vi "PreCalc FDFrame Durations.vi"(8 "error in (no error)":errorcluster, 9 "Bit Time FD (seconds)":dbl, 10 "Bit Time (seconds)":dbl, 11 "CANBus_Load_Calculator in":refnum<class "CANBus_Load_Calculator.lvclass">) -> (0 "error out":errorcluster, 3 "CANBus_Load_Calculator out":refnum<class "CANBus_Load_Calculator.lvclass">)   [LabVIEW 2018, in "NI-XNET Monitor Engine.lvlib" / "XNET-Bus-Load-Calculator.lvlib" / "CANBus_Load_Calculator.lvclass"]
uses:
  CANBus_Load_Calculator.lvclass
  typedefs/CANFD_Frame_Timing.ctl
  CANBus_Load_Calculator.lvclass/CANBus_Load_Calculator.ctl
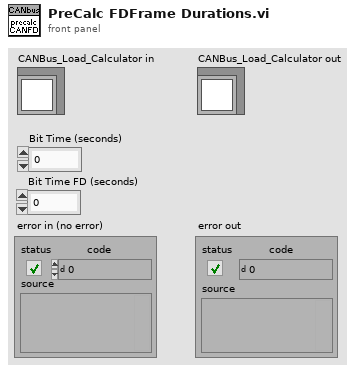
[diagram p1: front panel]
types:
  T1 = typedef "NI-XNET Monitor Engine.lvlib/XNET-Bus-Load-Calculator.lvlib/CANBus_Load_Calculator.lvclass/CANFD_Frame_Timing.ctl" = cluster{"Frame Length (Bytes)":i32, "FD.StdID.AvgDuration (us)":u32, "FD.ExtID.AvgDuration (us)":u32, "FDBRS.StdID.AvgDuration (us)":u32, "FDBRS.ExtID.AvgDuration (us)":u32}
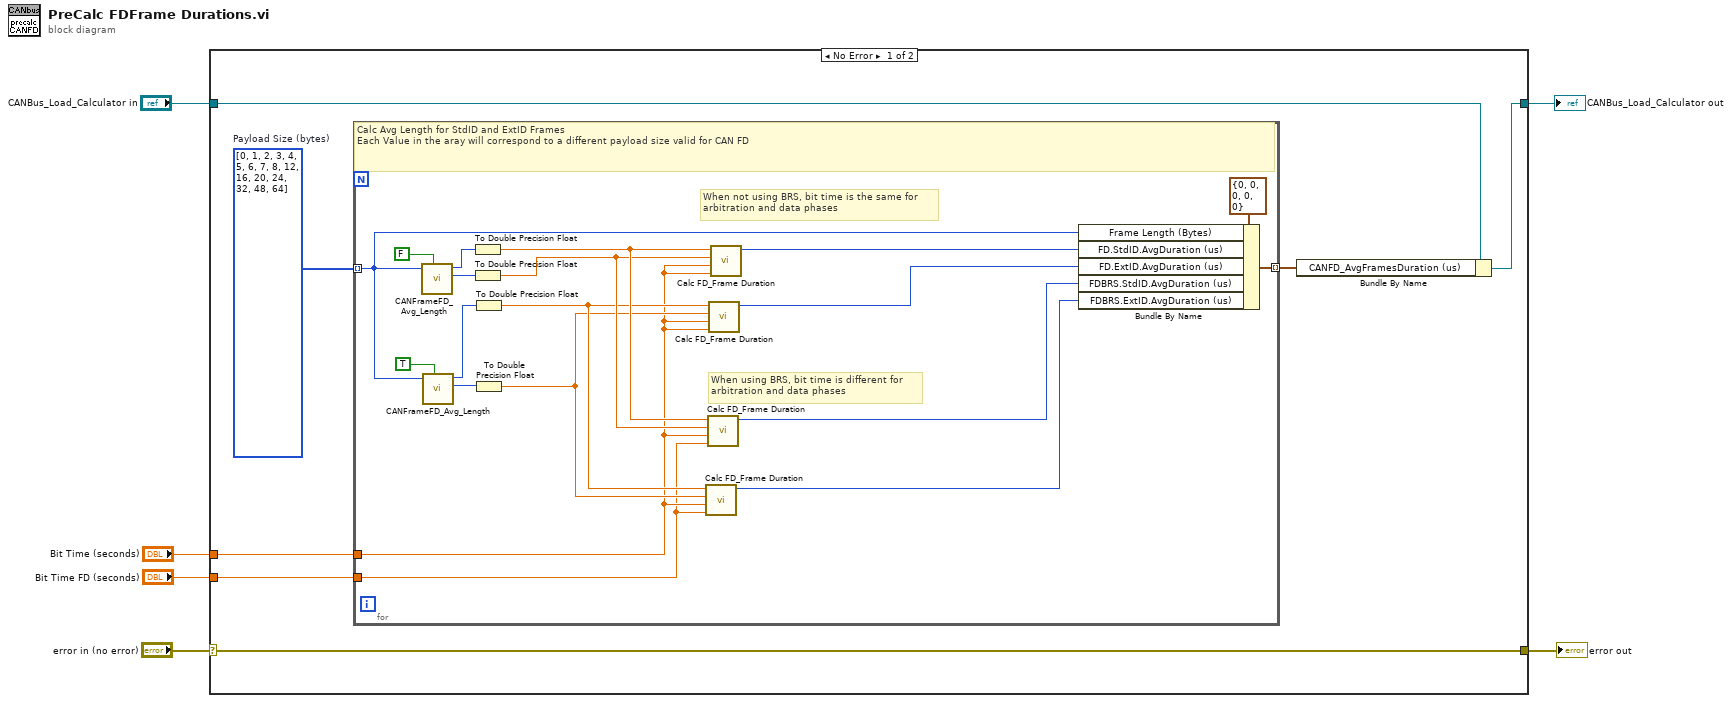
[diagram p0: block diagram]
diagram:
  n1 = case shown="No Error" "error in (no error)" {
    selector: "error in (no error)" -> [w11 w34]
    tunnel: "Bit Time (seconds)" -> [w9 _]
    tunnel: [w13 w33] -> w5
    tunnel: "CANBus_Load_Calculator in" -> [w12 w33]
    tunnel: [w11 w34] -> w2
    tunnel: "Bit Time FD (seconds)" -> [w8 _]
    frame No Error {
      w10 = i32[] [0, 1, 2, 3, 4, 5, 6, 7, 8, 12, 16, 20, 24, 32, 48, 64]  # Payload Size (bytes)
      n2 = for {
        tunnel: w10 -> [w28] mode=indexing
        tunnel: w9 -> [w15]
        tunnel: w8 -> [w14]
        tunnel: [w29] -> w7 mode=indexing
        # "When not using BRS, bit time is the same for\narbitration and data phases"
        # "When using BRS, bit time is different for\narbitration and data phases"
        # "Calc Avg Length for StdID and ExtID Frames\nEach Value in the aray will correspond to a different payload size valid for CAN FD"
        n3 = call "CANFrameFD_Avg_Length.vi"("Payload Size (bytes)"=w28, "Extended ID?"=FALSE) -> ("Avg.ArbitrationLength (bits)"=w27:i32, "Avg.DataLength (bits)"=w26:i32)  [unwired: 5 in]
        n4 = call "CANFrameFD_Avg_Length.vi"("Payload Size (bytes)"=w28, "Extended ID?"=TRUE) -> ("Avg.ArbitrationLength (bits)"=w25:i32, "Avg.DataLength (bits)"=w24:i32)  [unwired: 5 in]
        n5 = To Double Precision Float(number=w27) -> (double precision float=w21:dbl)
        n6 = To Double Precision Float(number=w26) -> (double precision float=w20:dbl)
        n7 = To Double Precision Float(number=w25) -> (double precision float=w19:dbl)
        n8 = To Double Precision Float(number=w24) -> (double precision float=w18:dbl)
        n9 = call "Calc FD_Frame Duration.vi"("Bit Time FD (seconds)"=w14, "Bit Time (seconds)"=w15, "Avg.DataLength (bits)"=w18, "Avg.ArbitrationLength (bits)"=w19) -> ("Frame.Duration(us)"=w23:u32)  [unwired: 7 in]
        n10 = call "Calc FD_Frame Duration.vi"("Bit Time FD (seconds)"=w14, "Bit Time (seconds)"=w15, "Avg.DataLength (bits)"=w20, "Avg.ArbitrationLength (bits)"=w21) -> ("Frame.Duration(us)"=w17:u32)  [unwired: 7 in]
        n11 = call "Calc FD_Frame Duration.vi"("Bit Time FD (seconds)"=w15, "Bit Time (seconds)"=w15, "Avg.DataLength (bits)"=w18, "Avg.ArbitrationLength (bits)"=w19) -> ("Frame.Duration(us)"=w16:u32)  [unwired: 7 in]
        n12 = call "Calc FD_Frame Duration.vi"("Bit Time FD (seconds)"=w15, "Bit Time (seconds)"=w15, "Avg.DataLength (bits)"=w20, "Avg.ArbitrationLength (bits)"=w21) -> ("Frame.Duration(us)"=w22:u32)  [unwired: 7 in]
        n13 = Bundle By Name(cluster=T1 {"Frame Length (Bytes)"=0, "FD.StdID.AvgDuration (us)"=0, "FD.ExtID.AvgDuration (us)"=0, "FDBRS.StdID.AvgDuration (us)"=0, "FDBRS.ExtID.AvgDuration (us)"=0} ("CANFD_Frame_Timing"), "Frame Length (Bytes)"=w28, "FD.StdID.AvgDuration (us)"=w22, "FD.ExtID.AvgDuration (us)"=w16, "FDBRS.StdID.AvgDuration (us)"=w17, "FDBRS.ExtID.AvgDuration (us)"=w23) -> (w29:T1)
      }
      n14 = Bundle By Name(cluster=w12, "CANFD_AvgFramesDuration (us)"=w7) -> (w13:refnum<class "CANBus_Load_Calculator.lvclass">)
    }
    frame Error {
    }
  }
  "CANBus_Load_Calculator out" <- w5
  "error out" <- w2
